vi "_CheckPrivilege.vi"(8 "error in":errorcluster, 11 "Privilege:":T1) -> (0 "error out":errorcluster, 2 "valid？":bool)   [LabVIEW 2017, in "Login-UI.lvlib"]
uses:
  Login-UI.lvlib
  User-Role.ctl
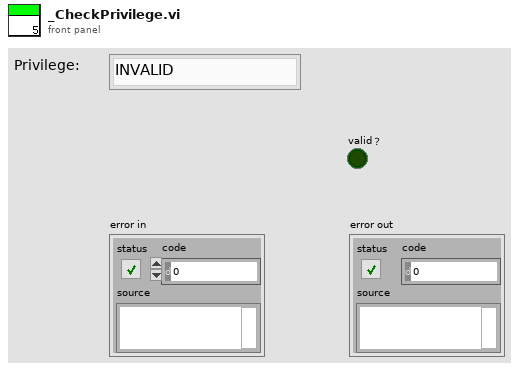
[diagram p1: front panel]
types:
  T1 = typedef "Login-UI.lvlib/User-Role.ctl" = enum16{"INVALID", "Operator", "Engineer", "Admin"}
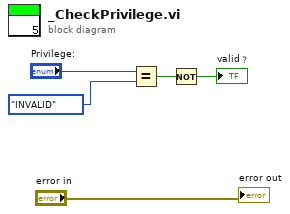
[diagram p0: block diagram]
diagram:
  n1 = Equal?(x="Privilege:", y=User-Role."INVALID" ("Privilege:")) -> (x = y?=w3:bool)
  n2 = Not(x=w3) -> (.not. x?=→"valid？":bool)
  "error out" <- "error in"
